vi "Get About Info.vi"(8 "error in":errorcluster, 11 "Lv Proj Document Type:TAF Proj":refnum<class "TAF Proj.lvclass">) -> (0 "error out":errorcluster, 3 "About":string)   [LabVIEW 2021, in "TAF Proj Document Type.lvlib" / "TAF Proj.lvclass"]
doc: "Overide this function to specify about info of your plugin.\n\nNote: These inforamtion are displayed in the Antidoc's About window."
uses:
  <vilib>/Wovalab/AntiDoc/Document Type/Add-ons/LabVIEW TAF Project/TAF Proj/TAF Proj.lvclass
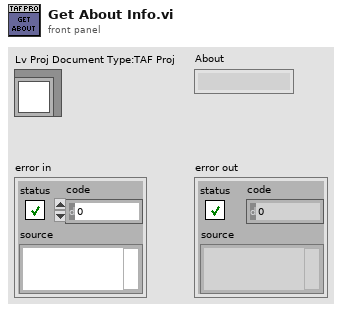
[diagram p1: front panel]
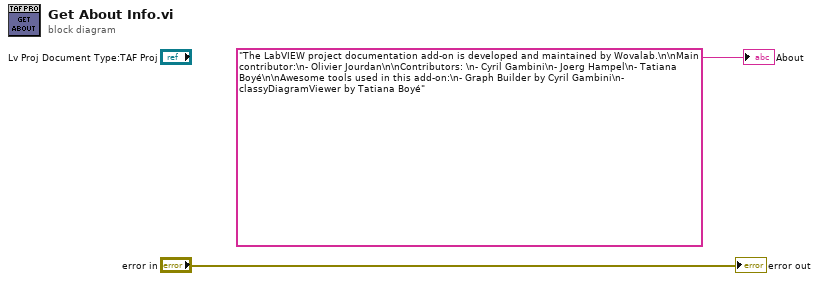
[diagram p0: block diagram]
diagram:
  "error out" <- "error in"
  "About" <- "The LabVIEW project documentation add-on is developed and maintained by Wovalab.\n\nMain contributor:\n- Olivier Jourdan\n\nContributors: \n- Cyril Gambini\n- Joerg Hampel\n- Tatiana Boyé\n\nAwesome tools used in this add-on:\n- Graph Builder by Cyril Gambini\n- classyDiagramViewer by Tatiana Boyé" ("About")
